vi "GetWIPDataWithOpenDB.vi"(8 "error in (no error)":errorcluster, 10 "Lotno":string, 11 "connection reference":T1) -> (0 "error out":errorcluster, 1 "step":string, 2 "data":i32, 3 "connection reference 2":T1, 4 "location":string, 6 "status":string)   [LabVIEW 2012]
uses:
  <vilib>/addons/database/Connection.llb/Conn ObjectReference.ctl
  <vilib>/addons/database/Auxilliary.llb/DB Tools Cursor Type.ctl
  <vilib>/addons/database/Connection.llb/Conn Execute.vi
  <vilib>/addons/database/Recordset.llb/Rec Fetch Integer Data (R).vi
  <vilib>/addons/database/Recordset.llb/Rec Destroy - Connection.vi
  <vilib>/addons/database/Recordset.llb/Rec Fetch Recordset Data (R).vi
  <vilib>/addons/database/_DB Variant To Data/Database Variant To Data.xnode
  <vilib>/addons/database/NI_Database_API.lvlib
panel:
  out "lotno":string
  out "Package":string
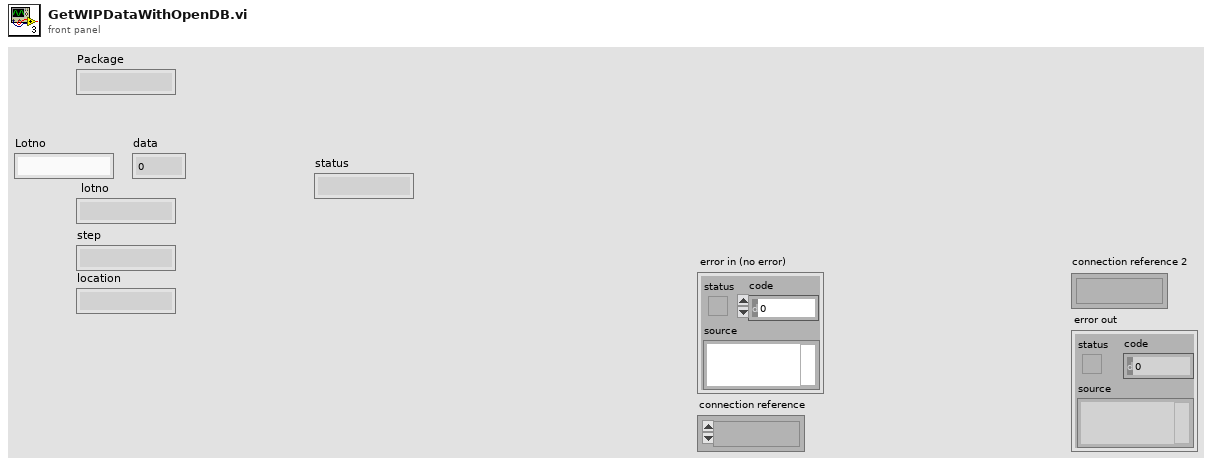
[diagram p1: front panel]
types:
  T1 = typedef "NI_Database_API.lvlib/Conn ObjectReference.ctl" = refnum<k1>
  T2 = typedef "NI_Database_API.lvlib/DB Tools Cursor Type.ctl" = enum16{"forward-only", "keyset", "dynamic", "static"}
  T3 = typedef "NI_Database_API.lvlib/Rec ObjectReference.ctl" = refnum<k1>
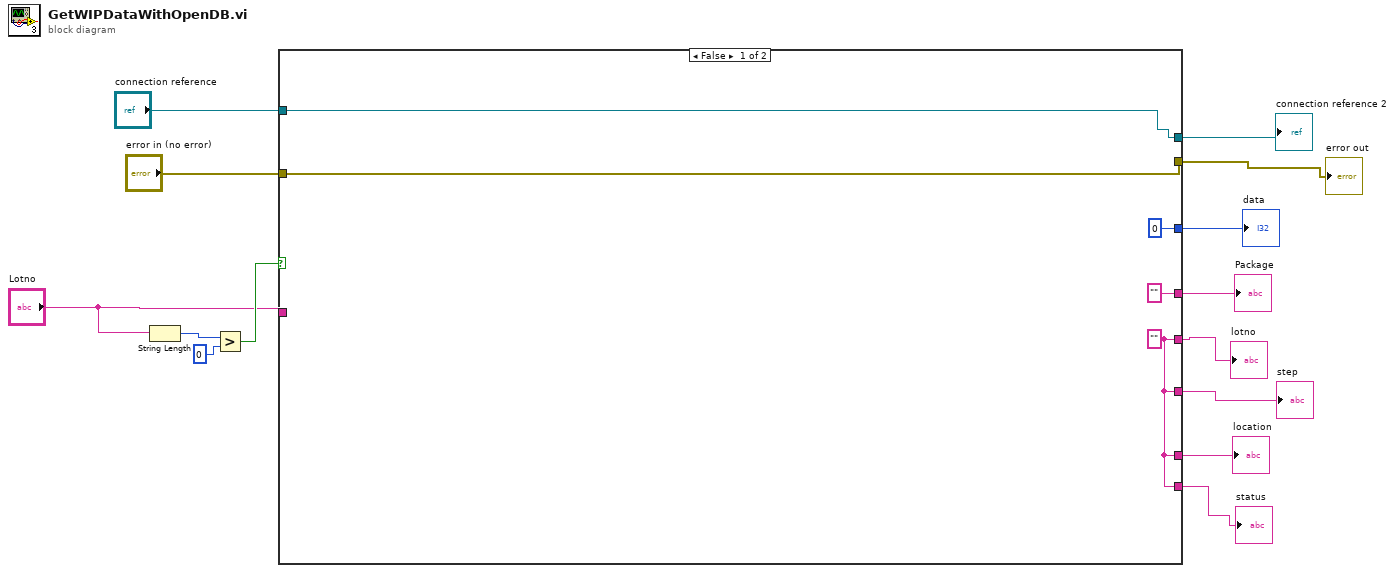
[diagram p0: block diagram]
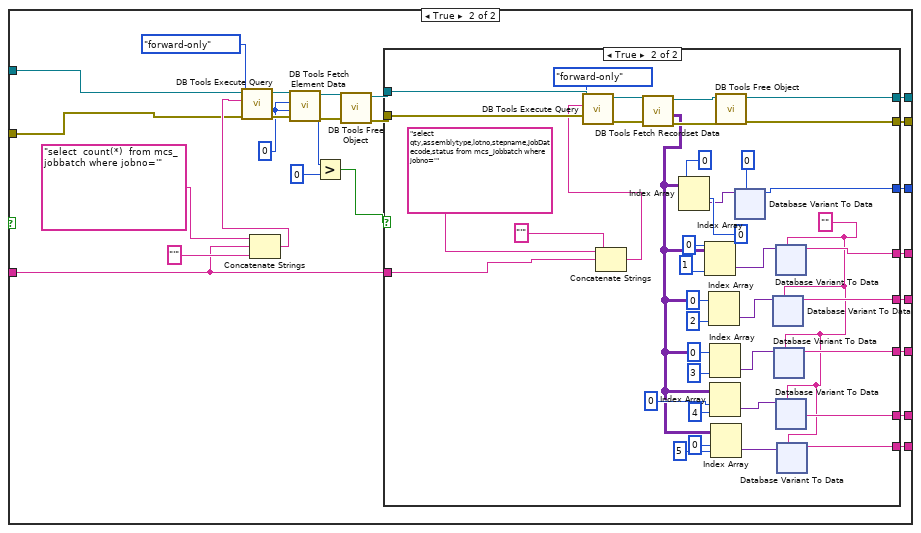
[diagram p2: hidden frame]
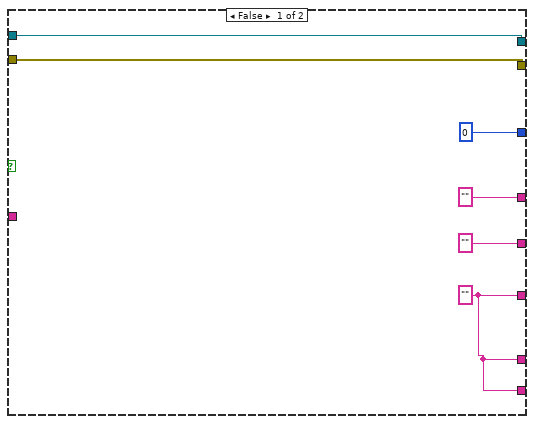
[diagram p3: hidden frame]
diagram:
  n1 = String Length(string="Lotno") -> (length=w14:i32)
  n2 = Greater?(x=w14, y=0) -> (0:w12:bool)
  n3 = case shown="False" w12 {
    tunnel: "Lotno" -> [_ w36]
    tunnel: [w15 w44] -> w11
    tunnel: ["" ("data") w43] -> w10
    tunnel: [0 ("data") w42] -> w9
    tunnel: [w15 w41] -> w8
    tunnel: [w15 w25] -> w7
    tunnel: "error in (no error)" -> [w16 w24]
    tunnel: "connection reference" -> [w17 w23]
    tunnel: [w17 w22] -> w4
    tunnel: [w16 w21] -> w3
    tunnel: [w15 w20] -> w2
    frame False {
      w15 = "" ("data")
    }
    frame True {
      w29 = 0
      n4 = Concatenate Strings("select  count(*)  from mcs_jobbatch where jobno='" ("string"), w36, "'" ("string")) -> (w34:string)
      n5 = call-poly <vilib>:"DB Tools Execute Query.vi"("error in (no error)"=w24, "cursor type"=DB_Tools_Cursor_Type."forward-only", "SQL query"=w34, "connection reference"=w23) -> ("error out"=w33:errorcluster, "recordset reference"=w32:T3)  [unwired: 4 in]
      n6 = call-poly <vilib>:"DB Tools Fetch Element Data.vi"("error in (no error)"=w33, "type"=w29, "column index"=w29, "recordset reference"=w32) -> ("error out"=w30:errorcluster, "data"=w28:i32, "recordset reference out"=w31:T3)  [unwired: 3 in]
      n7 = Greater?(x=w28, y=0) -> (0:w26:bool)
      n8 = call-poly <vilib>:"DB Tools Free Object.vi"("error in (no error)"=w30, "recordset reference"=w31) -> ("error out"=w39:errorcluster, "connection reference"=w40:T1)  [unwired: 8 in]
      n9 = case shown="True" w26 {
        tunnel: w40 -> [w47 w90]
        tunnel: w39 -> [w46 w87]
        tunnel: w36 -> [_ w70]
        tunnel: ["" ("data") w69] -> w44
        tunnel: ["" ("data") w68] -> w43
        tunnel: [0 ("data") w67] -> w42
        tunnel: [w45 w63] -> w41
        tunnel: [w45 w61] -> w25
        tunnel: [w47 w60] -> w22
        tunnel: [w46 w59] -> w21
        tunnel: [w45 w51] -> w20
        frame False {
          w45 = "" ("data")
        }
        frame True {
          w52 = ""
          n10 = Concatenate Strings("select qty,assemblytype,lotno,stepname,jobDatecode,status from mcs_jobbatch where jobno='" ("string"), w70, "'" ("string")) -> (w81:string)
          n11 = call-poly <vilib>:"DB Tools Execute Query.vi"("error in (no error)"=w87, "cursor type"=DB_Tools_Cursor_Type."forward-only", "SQL query"=w81, "connection reference"=w90) -> ("error out"=w86:errorcluster, "recordset reference"=w89:T3)  [unwired: 4 in]
          n12 = call-poly <vilib>:"DB Tools Fetch Recordset Data.vi"("error in (no error)"=w86, "recordset reference"=w89) -> ("error out"=w85:errorcluster, "recordset data"=w56:variant[][], "recordset reference out"=w88:T3)  [unwired: 3 in]
          n13 = Index Array(array=w56, index (row)=0, index (col)=0 ("disabled index (col)")) -> (element=w78:variant)
          n14 = Index Array(array=w56, index (row)=0 ("disabled index (row)"), index (col)=1 ("disabled index (col)")) -> (element=w74:variant)
          n15 = Index Array(array=w56, index (row)=0 ("disabled index (row)"), index (col)=2 ("disabled index (col)")) -> (element=w73:variant)
          n16 = Index Array(array=w56, index (row)=0 ("disabled index (row)"), index (col)=3 ("disabled index (col)")) -> (element=w64:variant)
          n17 = Index Array(array=w56, index (row)=0, index (col)=4 ("disabled index (col)")) -> (element=w62:variant)
          n18 = Index Array(array=w56, index (row)=0, index (col)=5 ("disabled index (col)")) -> (element=w53:variant)
          n19 = call-poly <vilib>:"DB Tools Free Object.vi"("error in (no error)"=w85, "recordset reference"=w88) -> ("error out"=w59:errorcluster, "connection reference"=w60:T1)  [unwired: 8 in]
          n20 = xnode "Database Variant To Data"("database variant"=w78, "type"=0) -> ("data"=w67:i32)  [unwired: 1 in, 1 out]
          n21 = xnode "Database Variant To Data"("database variant"=w73, "type"=w52) -> ("data"=w69:string)  [unwired: 1 in, 1 out]
          n22 = xnode "Database Variant To Data"("database variant"=w64, "type"=w52) -> ("data"=w63:string)  [unwired: 1 in, 1 out]
          n23 = xnode "Database Variant To Data"("database variant"=w74, "type"=w52) -> ("data"=w68:string)  [unwired: 1 in, 1 out]
          n24 = xnode "Database Variant To Data"("database variant"=w62, "type"=w52) -> ("data"=w61:string)  [unwired: 1 in, 1 out]
          n25 = xnode "Database Variant To Data"("database variant"=w53, "type"=w52) -> ("data"=w51:string)  [unwired: 1 in, 1 out]
        }
      }
    }
  }
  "data" <- w9
  "Package" <- w10
  "lotno" <- w11
  "step" <- w8
  "location" <- w7
  "connection reference 2" <- w4
  "error out" <- w3
  "status" <- w2
